vi "MGCC_FntStaMach_Initialization.vi"   [LabVIEW 2016]
doc: "-----------------------------------------------------------------------------------------------------------------------\nCopyright <2019> <The University of Tennessee at Knoxville and the University of Tennessee Research Foundation>\nThis software is released under BSD-3 \nhttps://opensource.org/licenses/BSD-3-Clause \nAdditional license options available at https://utrf.tennessee.edu/industry/sample-agreements/\n-----------------------------------------------------------------------------------------------------------------------\n\nThis VI is used to initize the events and flags in the FSM. In the future, it may be used to initize the variables in other function VIs."
uses:
  <vilib>/Utility/error.llb/Error Cluster From Error Code.vi
  MGCC_FntStaMach_gobal.vi
  <vilib>/ErrorRing/Error Ring.xnode
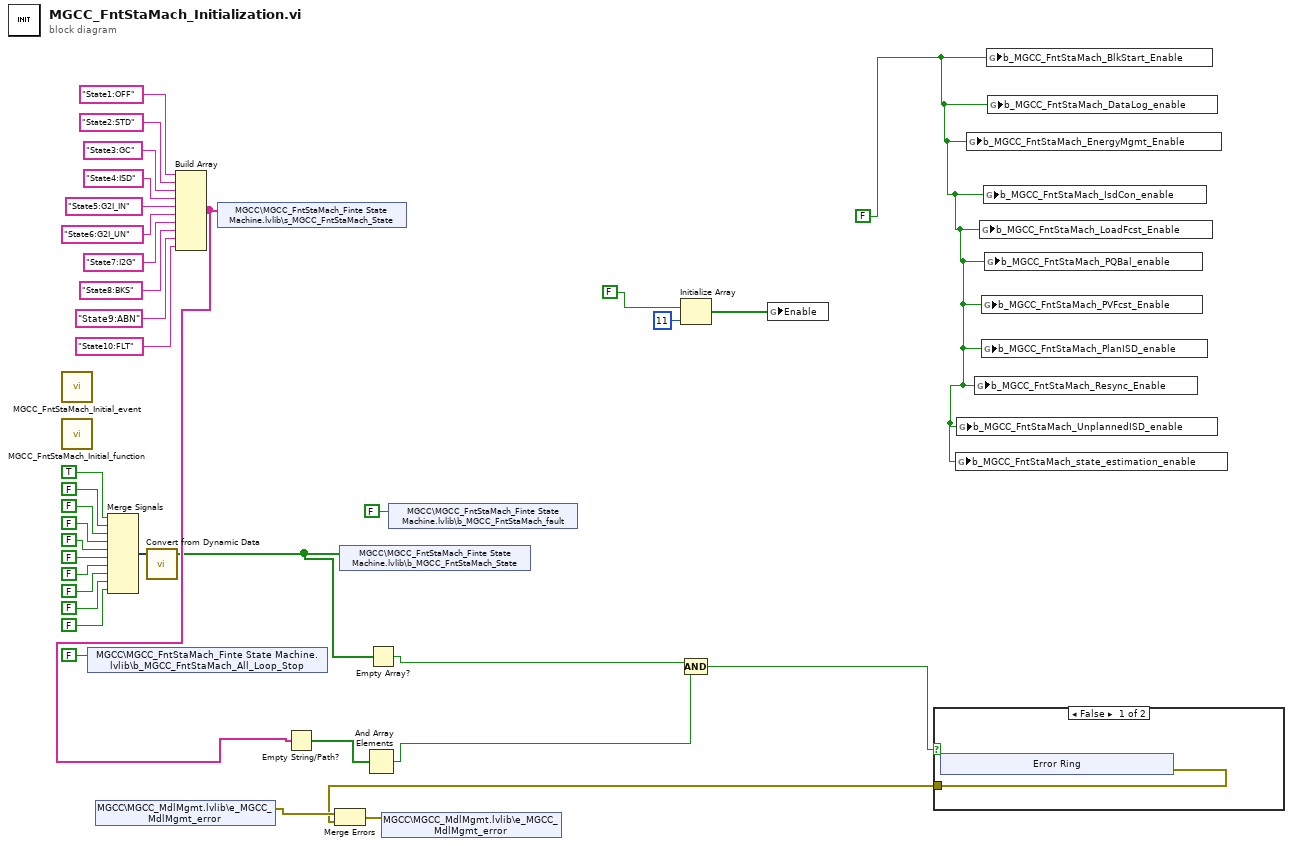
[diagram p0: block diagram]
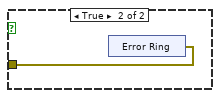
[diagram p2: hidden frame]
diagram:
  w1 = FALSE
  n1 = call "MGCC_FntStaMach_Initial_event.vi"() -> ()  [unwired: 12 in]
  n2 = call "MGCC_FntStaMach_Initial_function.vi"() -> ()  [unwired: 12 in]
  n3 = shared-variable "MGCC\\MGCC_FntStaMach_Finte State Machine.lvlib\\b_MGCC_FntStaMach_All_Loop_Stop"(FALSE ("ALL loop stop")) -> ()  [unwired: 1 in, 1 out]
  n4 = shared-variable "MGCC\\MGCC_MdlMgmt.lvlib\\e_MGCC_MdlMgmt_error"() -> (w13:errorcluster)  [unwired: 1 in, 1 out]
  n5 = Merge Signals(TRUE ("State3"), FALSE ("State3"), FALSE ("State3"), FALSE ("State3"), FALSE ("State3"), FALSE ("State3"), FALSE ("State3"), FALSE ("State3"), FALSE ("State3"), FALSE ("State3")) -> (w26:dynamicdata)
  n6 = call "Convert from Dynamic Data"("Dynamic Data Type"=w26) -> ("Array"=w7:bool[])  [unwired: 3 in]
  n7 = Build Array("State1:OFF", "State2:STD", "State3:GC", "State4:ISD", "State5:G2I_IN", "State6:G2I_UN", "State7:I2G", "State8:BKS", "State9:ABN", "State10:FLT") -> (w9:string[])
  n8 = shared-variable "MGCC\\MGCC_FntStaMach_Finte State Machine.lvlib\\s_MGCC_FntStaMach_State"(w9) -> ()  [unwired: 1 in, 1 out]
  n9 = Empty String/Path?(string/path=w9) -> (empty?=w8:bool[])
  n10 = shared-variable "MGCC\\MGCC_FntStaMach_Finte State Machine.lvlib\\b_MGCC_FntStaMach_State"(w7) -> ()  [unwired: 1 in, 1 out]
  n11 = And Array Elements(Boolean array=w8) -> (logical AND=w10:bool)
  n12 = Empty Array?(array=w7) -> (empty?=w6:bool)
  n13 = shared-variable "MGCC\\MGCC_FntStaMach_Finte State Machine.lvlib\\b_MGCC_FntStaMach_fault"(FALSE ("b_MGCC_FntStaMach_fault")) -> ()  [unwired: 1 in, 1 out]
  n14 = Initialize Array(FALSE, 11 ("dimension size")) -> (w2:bool[])
  n15 = Compound Arithmetic op=AND(w6, w10) -> (w5:bool)
  n16 = global write "MGCC_FntStaMach_gobal.vi" "Enable"(w2) -> ()
  n17 = case shown="False" w5 {
    tunnel: [w37 w43] -> w11
    frame False {
      n18 = xnode "Error Ring"() -> ("error out"=w37:errorcluster)
    }
    frame True {
      n19 = xnode "Error Ring"() -> ("error out"=w43:errorcluster)
    }
  }
  n20 = Merge Errors(w13, w11) -> (w12:errorcluster)
  n21 = shared-variable "MGCC\\MGCC_MdlMgmt.lvlib\\e_MGCC_MdlMgmt_error"(w12) -> ()  [unwired: 1 in, 1 out]
  n22 = global write "MGCC_FntStaMach_gobal.vi" "b_MGCC_FntStaMach_state_estimation_enable"(w1) -> ()
  n23 = global write "MGCC_FntStaMach_gobal.vi" "b_MGCC_FntStaMach_UnplannedISD_enable"(w1) -> ()
  n24 = global write "MGCC_FntStaMach_gobal.vi" "b_MGCC_FntStaMach_EnergyMgmt_Enable"(w1) -> ()
  n25 = global write "MGCC_FntStaMach_gobal.vi" "b_MGCC_FntStaMach_Resync_Enable"(w1) -> ()
  n26 = global write "MGCC_FntStaMach_gobal.vi" "b_MGCC_FntStaMach_LoadFcst_Enable"(w1) -> ()
  n27 = global write "MGCC_FntStaMach_gobal.vi" "b_MGCC_FntStaMach_PVFcst_Enable"(w1) -> ()
  n28 = global write "MGCC_FntStaMach_gobal.vi" "b_MGCC_FntStaMach_PlanISD_enable"(w1) -> ()
  n29 = global write "MGCC_FntStaMach_gobal.vi" "b_MGCC_FntStaMach_IsdCon_enable"(w1) -> ()
  n30 = global write "MGCC_FntStaMach_gobal.vi" "b_MGCC_FntStaMach_PQBal_enable"(w1) -> ()
  n31 = global write "MGCC_FntStaMach_gobal.vi" "b_MGCC_FntStaMach_BlkStart_Enable"(w1) -> ()
  n32 = global write "MGCC_FntStaMach_gobal.vi" "b_MGCC_FntStaMach_DataLog_enable"(w1) -> ()
